vi "Get String Occurences in 1D Array.vi"(9 "Search String":string, 11 "Array of Strings":string[](array[string])) -> (3 "# of Occurences":i32)   [LabVIEW 2024, in "Watlow F4T.lvclass"]
uses:
  Watlow F4T.lvclass
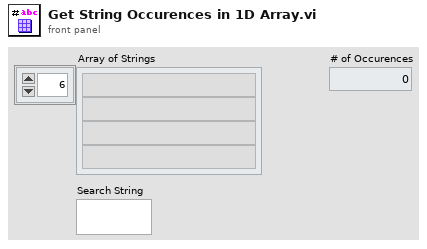
[diagram p1: front panel]
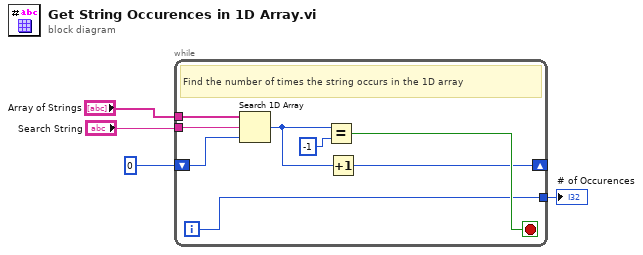
[diagram p0: block diagram]
diagram:
  n1 = while {
    tunnel: "Array of Strings" -> [w11]
    tunnel: "Search String" -> [w10]
    shift-right: [w6] -> _
    shift-left: 0 ("y") -> [w8]
    tunnel: [w5] -> w4
    i -> [w5]
    stop <- w9 stop-if-true
    # "Find the number of times the string occurs in the 1D array"
    n2 = Search 1D Array(1D array=w11, element=w10, start index (0)=w8) -> (index of element=w7:i32)
    n3 = Equal?(x=w7, y=-1) -> (x = y?=w9:bool)
    n4 = Increment(x=w7) -> (x+1=w6:i32)
  }
  "# of Occurences" <- w4
